vi "mfOvsfCodeGenerate.vi"(8 "error in (no error)":errorcluster caption="错误输入（无错误）", 9 "ovsf_No":dbl, 10 "sf":dbl, 11 "Path":path) -> (0 "error out":errorcluster caption="错误输出", 3 "ovsf_code":dbl[][](array[numeric]))   [LabVIEW 2015]
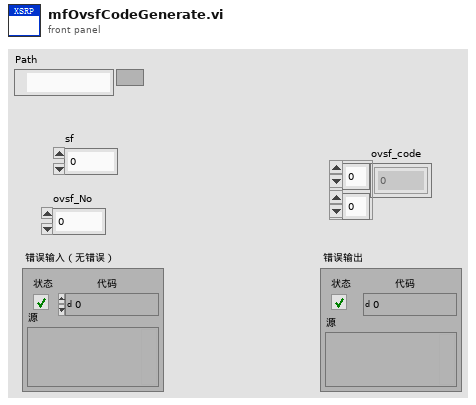
[diagram p1: front panel]
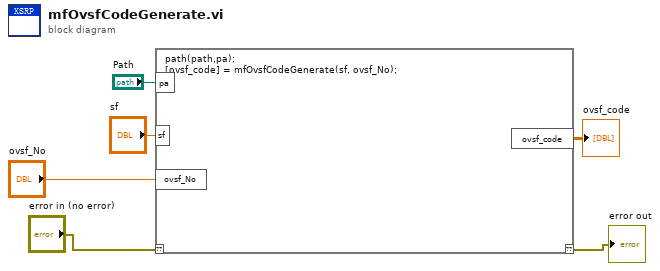
[diagram p0: block diagram]
diagram:
  n1 = script code="path(path,pa);\n[ovsf_code] = mfOvsfCodeGenerate(sf, ovsf_No);"("??"="error in (no error)", "pa"="Path", "sf"="sf", "ovsf_No"="ovsf_No") -> ("??"=→"error out":errorcluster, "ovsf_code"=→"ovsf_code":dbl[][])
